vi "window_graph init_interface.vi"(0 "XY Graph in":refnum<vi>, 1 "mouse event":refnum<vi>, 2 "Target plot":refnum<vi>, 3 "Area Plot":refnum<vi>, 11 "error in (no error)":errorcluster, 12 "plot name":string[](array[string]), 14 "shadow graph":refnum<vi>) -> (6 "refnum cluster output":T1, 15 "error out":errorcluster)   [LabVIEW 2018]
uses:
  <vilib>/Utility/miscctls.llb/LVPositionTypeDef.ctl
  mouse_state.ctl
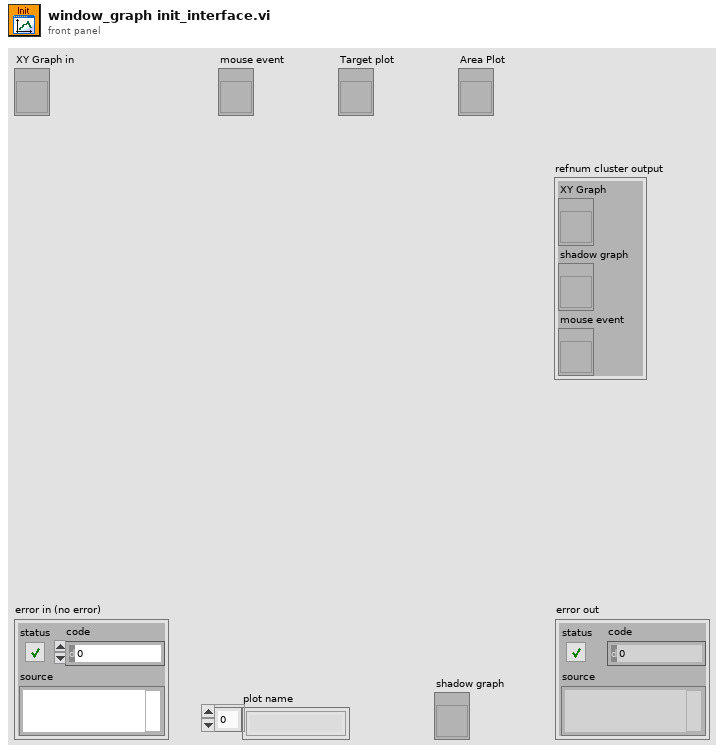
[diagram p1: front panel]
types:
  T1 = cluster{"XY Graph":refnum<vi>, "shadow graph":refnum<vi>, "mouse event":refnum<vi>}
  T2 = typedef "mouse_state.ctl" = enum16{"normal", "mouse down", "calc"}
  T3 = typedef "LVPositionTypeDef.ctl" = cluster{"Left":i32, "Top":i32}
  T4 = typedef "LVBoundsTypeDef.ctl" = cluster{"Width":u32, "Height":u32}
  T5 = typedef "LVRectTypeDef.ctl" = cluster{"Left":i16, "Top":i16, "Right":i16, "Bottom":i16}
  T6 = typedef "LVRangeTypeDef.ctl" = cluster{"Minimum":dbl, "Maximum":dbl, "Increment":dbl, "Minor Increment":dbl, "Start":dbl}
  T7 = cluster{"BGColor":u32, "GridX":bool, "GridY":bool, "LineColorArray":u32[], "LineWidthArray":u8[]}
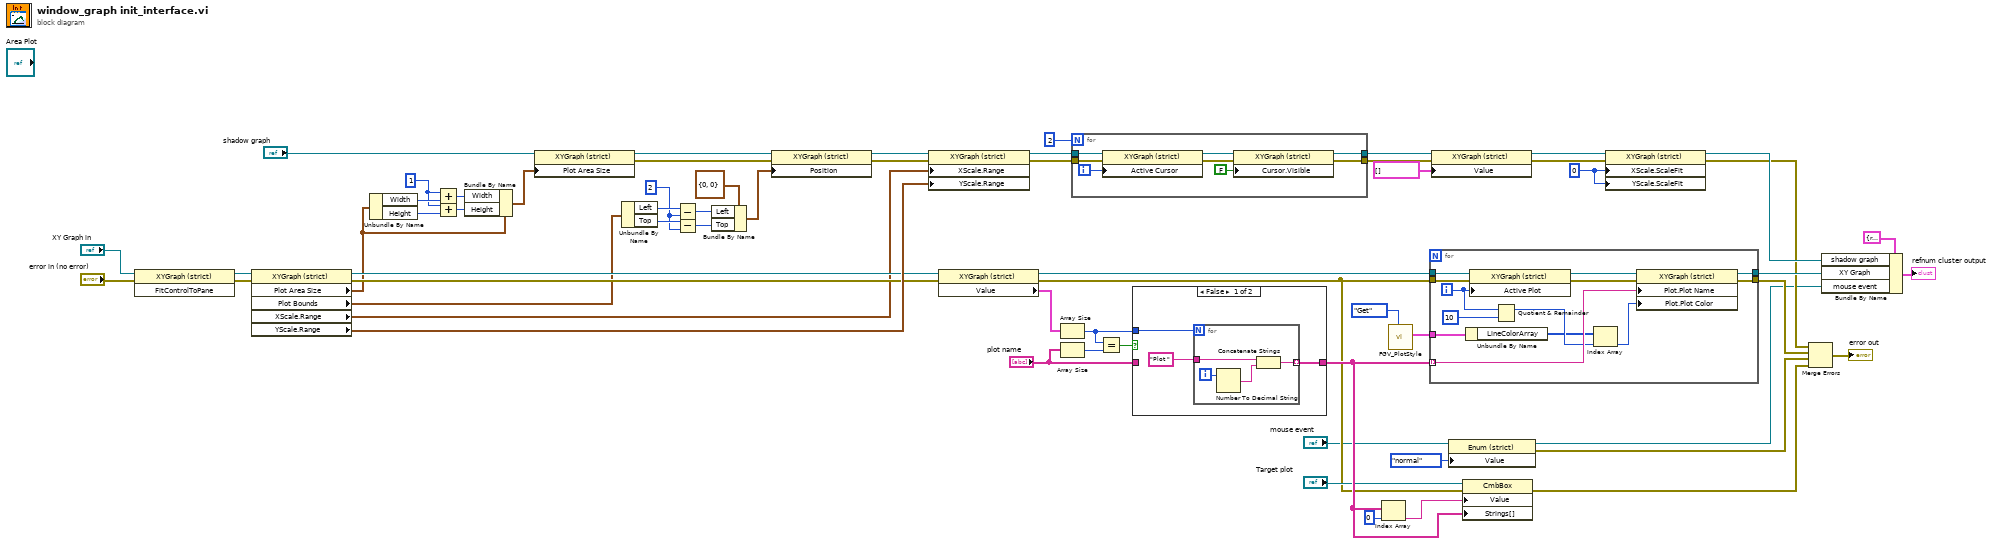
[diagram p0: block diagram]
diagram:
  w5 = u32 1 ("x")
  w10 = i16 2 ("x")
  w34 = u8 0 ("X Scale.Scale Fit")
  n1 = invoke class="XYGraph (strict)" method="FitControlToPane"(reference="XY Graph in", error in="error in (no error)") -> (reference out=w22:refnum<vi>, error out=w21:errorcluster)  [unwired: 1 in, 1 out]
  n2 = property class="XYGraph (strict)"(reference=w22, error in=w21) -> (reference out=w38:refnum<vi>, error out=w37:errorcluster, "Plot Area Size"=w1:T4, "Plot Bounds"=w14:T5, "XScale.Range"=w20:T6, "YScale.Range"=w61:T6)
  n3 = Unbundle By Name(w1) -> ("Width"=w7:u32, "Height"=w6:u32)
  n4 = Add(x=w5, y=w7) -> (x+y=w4:u32)
  n5 = Add(x=w5, y=w6) -> (x+y=w3:u32)
  n6 = Bundle By Name(cluster=w1, "Width"=w4, "Height"=w3) -> (w2:T4)
  n7 = property class="XYGraph (strict)"(reference="shadow graph", "Plot Area Size"=w2) -> (reference out=w19:refnum<vi>, error out=w18:errorcluster)  [unwired: 1 in]
  n8 = Unbundle By Name(w14) -> ("Left"=w12:i16, "Top"=w11:i16)
  n9 = Subtract(x=w12, y=w10) -> (x-y=w9:i16)
  n10 = Subtract(x=w11, y=w10) -> (x-y=w8:i16)
  n11 = Bundle By Name(cluster=T3 {"Left"=0, "Top"=0} ("Position"), "Left"=w9, "Top"=w8) -> (w15:T3)
  n12 = property class="XYGraph (strict)"(reference=w19, error in=w18, "Position"=w15) -> (reference out=w17:refnum<vi>, error out=w16:errorcluster)
  n13 = property class="XYGraph (strict)"(reference=w17, error in=w16, "XScale.Range"=w20, "YScale.Range"=w61) -> (reference out=w40:refnum<vi>, error out=w39:errorcluster)
  n14 = property class="XYGraph (strict)"(reference=w38, error in=w37) -> (reference out=w53:refnum<vi>, error out=w30:errorcluster, "Value"=w56:cluster{dbl[], sgl[]}[])
  n15 = Array Size(array=w56) -> (size(s)=w58:i32)
  n16 = Array Size(array="plot name") -> (size(s)=w60:i32)
  n17 = for {
    N: 2 -> [_]
    tunnel: w40 -> [w70]
    tunnel: [w65] -> w42
    tunnel: [w64] -> w41
    tunnel: w39 -> [w63]
    i -> [w69]
    n18 = property class="XYGraph (strict)"(reference=w70, error in=w63, "Active Cursor"=w69) -> (reference out=w68:refnum<vi>, error out=w67:errorcluster)
    n19 = property class="XYGraph (strict)"(reference=w68, error in=w67, "Cursor.Visible"=FALSE) -> (reference out=w65:refnum<vi>, error out=w64:errorcluster)
  }
  n20 = Equal?(x=w58, y=w60) -> (x = y?=w59:bool)
  n21 = case shown="False" w59 {
    tunnel: "plot name" -> [_ w78]
    tunnel: [w71 w78] -> w52
    tunnel: w58 -> [w72 _]
    frame False {
      n22 = for {
        N: w72 -> [_]
        tunnel: "Plot " -> [w76]
        tunnel: [w74] -> w71 mode=indexing
        i -> [w77]
        n23 = Number To Decimal String(number=w77) -> (decimal integer string=w75:string)  [unwired: 1 in]
        n24 = Concatenate Strings(w76, w75) -> (w74:string)
      }
    }
    frame True {
    }
  }
  n25 = Index Array(array=w52, index=0) -> (element=w54:string)
  n26 = call "FGV_PlotStyle.vi"("Function"=enum16{"Set", "Get"}."Get") -> ("Output Cluster"=w50:T7)  [unwired: 9 in, 1 out]
  n27 = for {
    tunnel: w52 -> [w87] mode=indexing
    tunnel: w53 -> [w91]
    tunnel: w30 -> [w90]
    tunnel: w50 -> [w85]
    tunnel: [w81] -> w48
    tunnel: [w79] -> w44
    i -> [w80]
    n28 = Unbundle By Name(w85) -> ("LineColorArray"=w83:u32[])
    n29 = property class="XYGraph (strict)"(reference=w91, error in=w90, "Active Plot"=w80) -> (reference out=w89:refnum<vi>, error out=w88:errorcluster)
    n30 = Quotient & Remainder(x=w80, y=10) -> (x-y*floor(x/y)=w86:i32)  [unwired: 1 out]
    n31 = Index Array(array=w83, index=w86) -> (element=w82:u32)
    n32 = property class="XYGraph (strict)"(reference=w89, error in=w88, "Plot.Plot Name"=w87, "Plot.Plot Color"=w82) -> (reference out=w79:refnum<vi>, error out=w81:errorcluster)
  }
  n33 = property class="XYGraph (strict)"(reference=w42, error in=w41, "Value"=cluster{"Array":cluster{"X":dbl, "Y":dbl}[]}[] []) -> (reference out=w36:refnum<vi>, error out=w35:errorcluster)
  n34 = property class="Enum (strict)"(reference="mouse event", "Value"=mouse_state."normal") -> (reference out=w26:refnum<vi>, error out=w27:errorcluster)  [unwired: 1 in]
  n35 = property class="CmbBox"(reference="Target plot", error in=w30, "Value"=w54, "Strings[]"=w52) -> (error out=w47:errorcluster)  [unwired: 1 out]
  n36 = property class="XYGraph (strict)"(reference=w36, error in=w35, "XScale.ScaleFit"=w34, "YScale.ScaleFit"=w34) -> (reference out=w33:refnum<vi>, error out=w32:errorcluster)
  n37 = Merge Errors(w32, w48, w27, w47) -> (→"error out":errorcluster)
  n38 = Bundle By Name(cluster=T1 {"XY Graph"=refnum, "shadow graph"=refnum, "mouse event"=refnum} ("refnum cluster output"), "shadow graph"=w33, "XY Graph"=w44, "mouse event"=w26) -> (→"refnum cluster output":T1)
